vi "LP MDrive init.vi"(0 "VISA IN":refnum<visa-resource-name>="COM17", 1 "Factory Default":bool, 5 "error in":errorcluster, 6 "Hold Current":string="50", 7 "Accel Setpoint":string="300000", 8 "Working Velocity":string, 9 "Mdrive Mode":T1=enum."Party Mode", 11 "Device Name":string, 12 "Run Current":string="50", 13 "Decel Setpoint":string="300000") -> (14 "VISA OUT":refnum<visa-resource-name>="COM17", 19 "error out":errorcluster)   [LabVIEW 2015]
uses:
  MCode_LV_86/Set Parameter.ctl
  MCode_LV_86/Get Parameter.ctl
  MCode_LV_86/MDrive Mode.ctl
panel:
  out "read buffer":string
  out "OK":bool
  out "Error":string
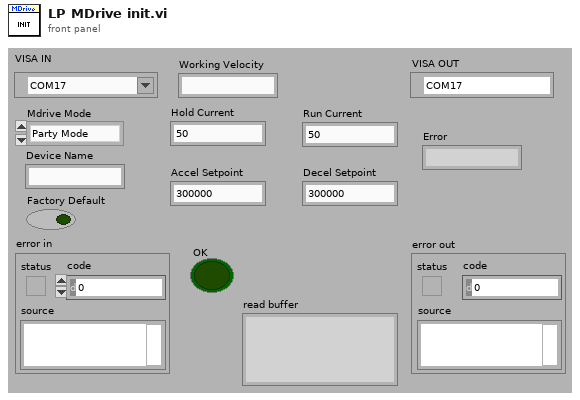
[diagram p1: front panel]
types:
  T1 = typedef "MDrive Mode.ctl" = enum16{"Normal Mode", "Party Mode"}
  T2 = typedef "Get Parameter.ctl" = enum16{"Acceleration (A)", "Baud Rate (BD)", "Busy Flag (BY)", "Counter 1 (C1)", "Counter 2 (C2)", "Check Sum Enable (CK)", "Clock Mode (CM)", "Clock Mode Ratio (CR)", "Clock Mode Out Step Width (CW)", "Deceleration (D)", "Digital Filtering, Input 1 (D1)", "Digital Filtering, Input 2 (D2)", "Digital Filtering, Input 3 (D3)", "Digital Filtering, Input 4 (D4)", "Digital Filtering, Input 5 (D5)", "Digital Filtering, Input 9 (D9)", "Digital Filtering, Input 10 (D10)", "Digital Filtering, Input 11 (D11)", "Digital Filtering, Input 12 (D12)", "Deadband (DB)", "Enable/Disable Drive (DE)", "Device Name (DN)", "End Program Execution (E)", "Encoder Function Enable (EE)", "Encoder Lines (EL)", "Error Flag (EF)", "Error Variable (ER)", "Echo Mode (EM)", "Escape (ES)", "Execute Program at Address (EX)", "Hold Current (HC)", "Hold Current Delay Time (HI)", "Input 1 (I1)", "Input 2 (I2)", "Input 3 (I3)", "Input 4 (I4)", "Input 5 Analog (I5)", "Input 6 Encoder Index (I6)", "Input 9 (I9)", "Input 10 (I10)", "Input 11 (I11)", "Input 12 (I12)", "Input Low Byte (1-4) (IL)", "Input High Byte (9-12) (IH)", "Inputs Total (1-4,9-12) (IN)", "Internal Temperature (IT)", "Jog Enable (JE)", "Limit Stop Mode (LM)", "MicroStepping Select (MS)", "Motor Settling Delay Time (MT)", "Moving Flag (MV)", "Output 1 (O1)", "Output 2 (O2)", "Output 3 (O3)", "Output 4 (O4)", "Output 9 (O9)", "Output 10 (O10)", "Output 11 (O11)", "Output 12 (O12)", "Output High Byte (9-12) (OH)", "Output Low Byte (1-4) (OL)", "Output Total (1-4 and 9-12) (OT)", "Position (P)", "Position Captured at Trip (PC)", "Position Maintenance (PM)", "Part Number (PN)", "Party Mode (PY)", "Register 1 (R1)", "Register 2 (R2)", "Register 3 (R3)", "Register 4 (R4)", "Run Current (RC)", "Serial Number (SN)", "Stall Flag (ST)", "Stall Factor (SF)", "Stall Mode Set (SM)", "User Variables (UV)", "Velocity (V)", "Velocity Changing Flag (VC)", "Velocity Initial (VI)", "Version, Firmware (VR)", "Velocity Maximum (VM)", "Read Input1", "Read Input2"}
  T3 = typedef "Set Parameter.ctl" = enum16{"Acceleration (A)", "Baud Rate (BD)", "Counter 1 (C1)", "Counter 2 (C2)", "Control C Software Reset (CE)", "Check Sum Enable (CK)", "Clock Mode (CM)", "Clock Mode Ratio (CR)", "Clock Mode Out Step Width (CW)", "Deceleration (D)", "Digital Filtering, Input 1 (D1)", "Digital Filtering, Input 2 (D2)", "Digital Filtering, Input 3 (D3)", "Digital Filtering, Input 4 (D4)", "Digital Filtering, Input 5 (D5)", "Digital Filtering, Input 9 (D9)", "Digital Filtering, Input 10 (D10)", "Digital Filtering, Input 11 (D11)", "Digital Filtering, Input 12 (D12)", "Deadband (DB)", "Decrement Variable (DC)", "Enable/Disable Drive (DE)", "Device Name (DN)", "End Program Execution (E)", "Encoder Function Enable (EE)", "Encoder Lines (EL)", "Echo Mode (EM)", "Error Clear (ER)", "Escape (ES)", "Execute Program at Address (EX)", "Factory Default (FD)", "Hold (H)", "Hold Current (HC)", "Hold Current Encoder Index (HI)", "Home to Home Switch (HM)", "Home to Delay Time (HT)", "Increment Variable (IC)", "Initialize Parameters to NVM (IP)", "Input into Variable (IV)", "Jog Enable (JE)", "Limit Stop Mode (LM)", "Move Absolute (MA)", "Move Relative (MR)", "MicroStepping Select (MS)", "Motor Settling Delay Time (MT)", "Output 1 (O1)", "Output 2 (O2)", "Output 3 (O3)", "Output 4 (O4)", "Output 9 (O9)", "Output 10 (O10)", "Output 11 (O11)", "Output 12 (O12)", "Output High Byte (9-12) (OH)", "Output Low Byte (1-4) (OL)", "Output Total (1-4 and 9-12) (OT)", "Position (P)", "Position Maintenance (PM)", "Party Mode (PY)", "Register 1 (R1)", "Register 2 (R2)", "Register 3 (R3)", "Register 4 (R4)", "Run Current (RC)", "Stall Factor (SF)", "Slew (SL)", "Stall Mode Set (SM)", "Upgrade Firmware (UG)", "Velocity Initial (VI)", "Velocity Maximum (VM)", "Set Input #1 as Home (S1)", "Save (S)", "Save DN+PY (NameS)", "Active Party Mode (0x0A)", "Set Input #1 (S1) as Limit- Active Floating", "Set Input #2 (S2) as Limit+ Active Floating", "Set Input #1 as Home (S1) Active Floating", "Set Input #1 as Home (S2) Active Floating", "Set Input #1 (S1) as Limit+ Active Floating", "Set Input #2 (S2) as Limit- Active Floating", "Hybrid Mode (AS)"}
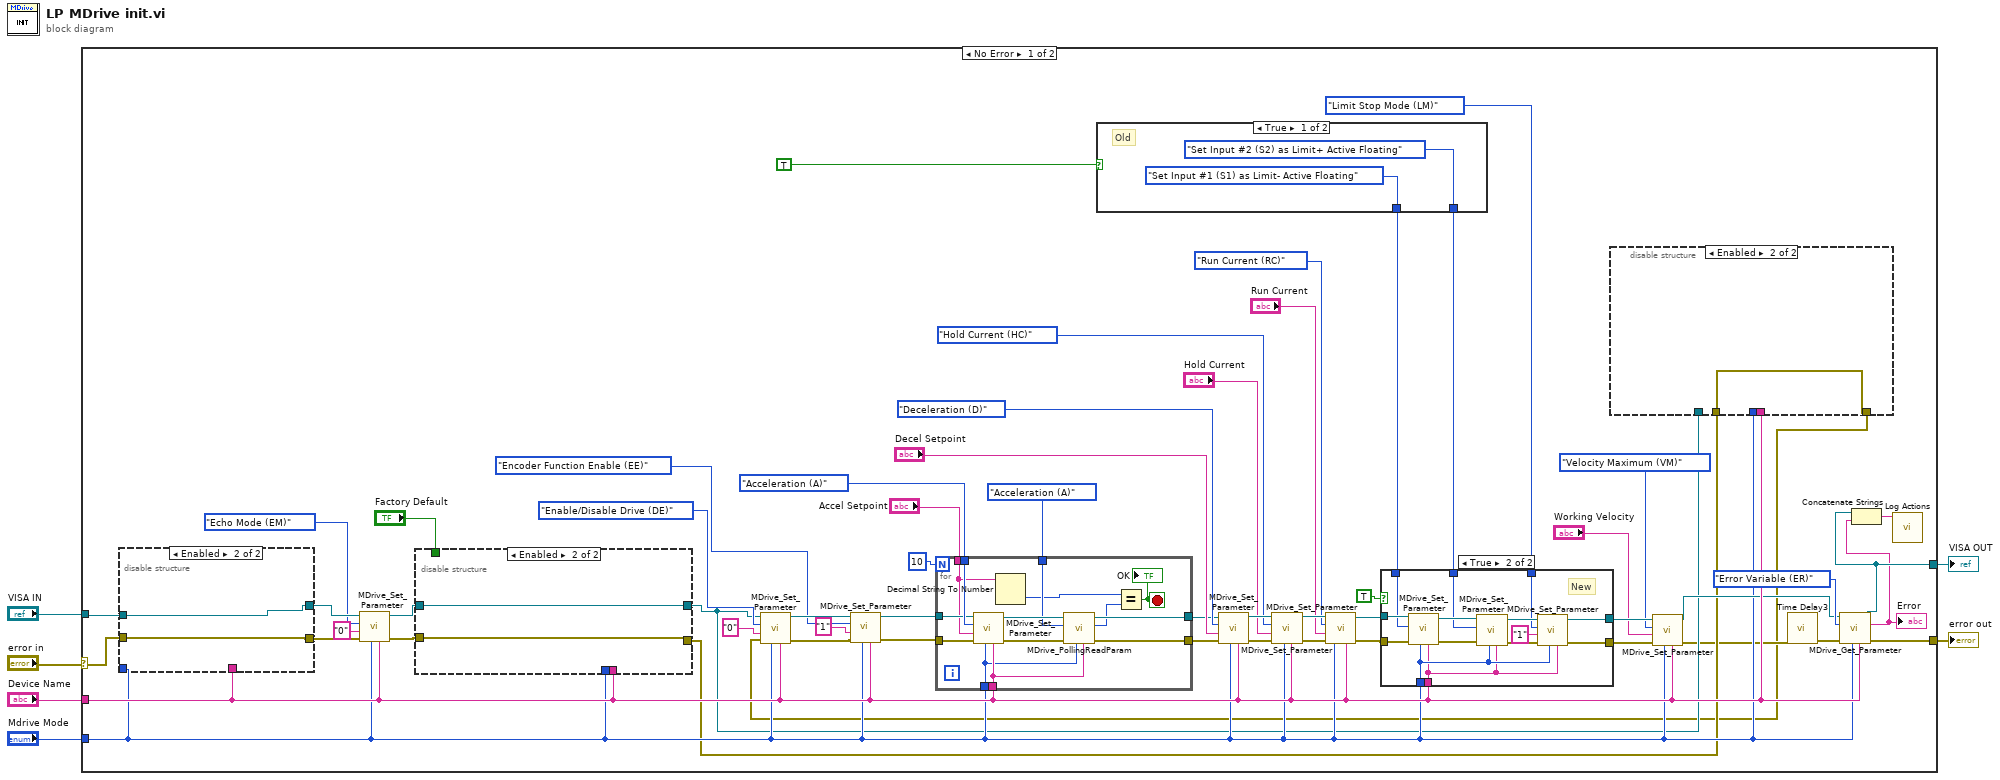
[diagram p0: block diagram]
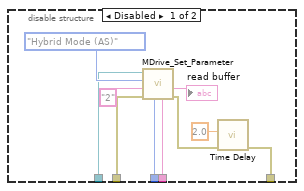
[diagram p2: hidden frame]
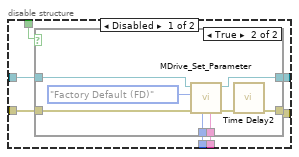
[diagram p3: hidden frame]
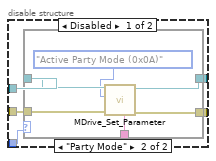
[diagram p5: hidden frame]
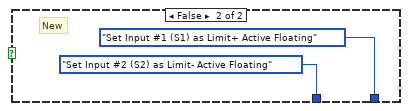
[diagram p7: hidden frame]
diagram:
  n1 = case shown="No Error" "error in" {
    selector: "error in" -> [w35 w145]
    tunnel: [w43 w144] -> w3
    tunnel: [w48 w145] -> w6
    tunnel: "VISA IN" -> [w36 w144]
    tunnel: "Device Name" -> [w13 _]
    tunnel: "Mdrive Mode" -> [w11 _]
    frame No Error {
      n2 = disable-structure shown="Enabled" {
        disable-tunnel: w36 -> [w113 w123]
        disable-tunnel: w35 -> [w112 w122]
        disable-tunnel: [w111 w123] -> w34
        disable-tunnel: [w110 w122] -> w33
        disable-tunnel: w13 -> [w109 _]
        disable-tunnel: w11 -> [w108 _]
        frame Disabled {
          n3 = case shown="\"Party Mode\"" w108 {
            tunnel: [w114 w121] -> w110
            tunnel: w112 -> [w114 w120]
            tunnel: [w115 w119] -> w111
            tunnel: w113 -> [w115 w118]
            tunnel: w109 -> [_ w116]
            frame "Normal Mode", Default {
            }
            frame "Party Mode" {
              n4 = call "MDrive_Set_Parameter.vi"("Device Name"=w116, "error in"=w120, "Set Parameter"=Set_Parameter."Active Party Mode (0x0A)", "VISA IN"=w118) -> ("error out"=w121:errorcluster, "VISA OUT"=w119:refnum<visa-resource-name>)  [unwired: 5 in, 1 out]
            }
          }
        }
        frame Enabled {
        }
      }
      n5 = call "MDrive_Set_Parameter.vi"("Device Name"=w13, "Mdrive Mode"=w11, "error in"=w33, "Parameter Setpoint"="0", "Set Parameter"=Set_Parameter."Echo Mode (EM)", "VISA IN"=w34) -> ("error out"=w32:errorcluster, "VISA OUT"=w31:refnum<visa-resource-name>)  [unwired: 3 in, 1 out]
      n6 = disable-structure shown="Enabled" {
        disable-tunnel: [w95 w106] -> w10
        disable-tunnel: [w94 w107] -> w9
        disable-tunnel: "Factory Default" -> [w93 _]
        disable-tunnel: w32 -> [w92 w106]
        disable-tunnel: w31 -> [w91 w107]
        disable-tunnel: w13 -> [w90 _]
        disable-tunnel: w11 -> [w89 _]
        frame Disabled {
          n7 = case shown="True" w93 {
            tunnel: [w96 w105] -> w95
            tunnel: w91 -> [w97 w104]
            tunnel: [w97 w103] -> w94
            tunnel: w92 -> [w96 w100]
            tunnel: w90 -> [_ w99]
            tunnel: w89 -> [_ w98]
            frame False {
            }
            frame True {
              n8 = call "MDrive_Set_Parameter.vi"("Device Name"=w99, "Mdrive Mode"=w98, "error in"=w100, "Set Parameter"=Set_Parameter."Factory Default (FD)", "VISA IN"=w104) -> ("error out"=w102:errorcluster, "VISA OUT"=w103:refnum<visa-resource-name>)  [unwired: 4 in, 1 out]
              n9 = call "Time Delay2"("error in (no error)"=w102) -> ("error out"=w105:errorcluster)  [unwired: 10 in]
            }
          }
        }
        frame Enabled {
        }
      }
      n10 = case shown="True" TRUE {
        tunnel: [Set_Parameter."Set Input #1 (S1) as Limit- Active Floating" ("Set Parameter") Set_Parameter."Set Input #2 (S2) as Limit- Active Floating" ("Set Parameter")] -> w41
        tunnel: [Set_Parameter."Set Input #2 (S2) as Limit+ Active Floating" ("Set Parameter") Set_Parameter."Set Input #1 (S1) as Limit+ Active Floating" ("Set Parameter")] -> w40
        frame True {
          # "Old"
        }
        frame False {
          # "New"
        }
      }
      n11 = disable-structure shown="Enabled" {
        disable-tunnel: w13 -> [w73 _]
        disable-tunnel: w11 -> [w72 _]
        disable-tunnel: w10 -> [w69 w74]
        disable-tunnel: w9 -> [w68 _]
        disable-tunnel: [w65 w74] -> w7
        frame Disabled {
          n12 = call "MDrive_Set_Parameter.vi"("Device Name"=w73, "Mdrive Mode"=w72, "error in"=w69, "Parameter Setpoint"="2", "Set Parameter"=Set_Parameter."Hybrid Mode (AS)", "VISA IN"=w68) -> ("error out"=w66:errorcluster, "read buffer"=→"read buffer":string)  [unwired: 3 in, 1 out]
          n13 = call "Time Delay"("error in (no error)"=w66, "Delay Time (s)"=2.0) -> ("error out"=w65:errorcluster)  [unwired: 9 in]
        }
        frame Enabled {
        }
      }
      n14 = call "MDrive_Set_Parameter.vi"("Device Name"=w13, "Mdrive Mode"=w11, "error in"=w7, "Parameter Setpoint"="0", "Set Parameter"=Set_Parameter."Enable/Disable Drive (DE)", "VISA IN"=w9) -> ("error out"=w17:errorcluster, "VISA OUT"=w18:refnum<visa-resource-name>)  [unwired: 3 in, 1 out]
      n15 = call "MDrive_Set_Parameter.vi"("Device Name"=w13, "Mdrive Mode"=w11, "error in"=w17, "Parameter Setpoint"="1", "Set Parameter"=Set_Parameter."Encoder Function Enable (EE)", "VISA IN"=w18) -> ("error out"=w16:errorcluster, "VISA OUT"=w15:refnum<visa-resource-name>)  [unwired: 3 in, 1 out]
      n16 = for {
        N: 10 -> [_]
        tunnel: "Accel Setpoint" -> [w77]
        tunnel: Set_Parameter."Acceleration (A)" ("Set Parameter") -> [w88]
        tunnel: w15 -> [w87]
        tunnel: w16 -> [w86]
        tunnel: [w83] -> w24
        tunnel: [w82] -> w23
        tunnel: Get_Parameter."Acceleration (A)" ("Get Parameter") -> [w81]
        tunnel: w13 -> [w80]
        tunnel: w11 -> [w79]
        stop <- w75 stop-if-true
        n17 = call "MDrive_Set_Parameter.vi"("Device Name"=w80, "Mdrive Mode"=w79, "error in"=w86, "Parameter Setpoint"=w77, "Set Parameter"=w88, "VISA IN"=w87) -> ("error out"=w84:errorcluster, "VISA OUT"=w85:refnum<visa-resource-name>)  [unwired: 3 in, 1 out]
        n18 = Decimal String To Number(string=w77) -> (number=w76:i32)  [unwired: 2 in, 1 out]
        n19 = call "MDrive_PollingReadParam.vi"("Device Name"=w80, "Mdrive Mode"=w79, "error in (no error)"=w84, "Get Parameter"=w81, "VISA Refnum in"=w85) -> ("error out"=w82:errorcluster, "Value"=w78:i32, "VISA Refnum out"=w83:refnum<visa-resource-name>)  [unwired: 3 in, 1 out]
        n20 = Equal?(x=w76, y=w78) -> (x = y?=w75:bool)
        "OK" <- w75
      }
      n21 = call "MDrive_Set_Parameter.vi"("Device Name"=w13, "Mdrive Mode"=w11, "error in"=w23, "Parameter Setpoint"="Decel Setpoint", "Set Parameter"=Set_Parameter."Deceleration (D)", "VISA IN"=w24) -> ("error out"=w60:errorcluster, "VISA OUT"=w61:refnum<visa-resource-name>)  [unwired: 3 in, 1 out]
      n22 = call "MDrive_Set_Parameter.vi"("Device Name"=w13, "Mdrive Mode"=w11, "error in"=w60, "Parameter Setpoint"="Hold Current", "Set Parameter"=Set_Parameter."Hold Current (HC)", "VISA IN"=w61) -> ("error out"=w58:errorcluster, "VISA OUT"=w59:refnum<visa-resource-name>)  [unwired: 3 in, 1 out]
      n23 = call "MDrive_Set_Parameter.vi"("Device Name"=w13, "Mdrive Mode"=w11, "error in"=w58, "Parameter Setpoint"="Run Current", "Set Parameter"=Set_Parameter."Run Current (RC)", "VISA IN"=w59) -> ("error out"=w19:errorcluster, "VISA OUT"=w20:refnum<visa-resource-name>)  [unwired: 3 in, 1 out]
      n24 = case shown="True" TRUE {
        tunnel: w20 -> [w129 w143]
        tunnel: w19 -> [w128 w142]
        tunnel: w11 -> [_ w131]
        tunnel: w13 -> [_ w130]
        tunnel: [w128 w134] -> w27
        tunnel: [w129 w135] -> w28
        tunnel: w41 -> [_ w139]
        tunnel: w40 -> [_ w138]
        tunnel: Set_Parameter."Limit Stop Mode (LM)" ("Set Parameter") -> [_ w133]
        frame False {
          # "OLD"
        }
        frame True {
          # "New"
          n25 = call "MDrive_Set_Parameter.vi"("Device Name"=w130, "Mdrive Mode"=w131, "error in"=w142, "Set Parameter"=w139, "VISA IN"=w143) -> ("error out"=w141:errorcluster, "VISA OUT"=w140:refnum<visa-resource-name>)  [unwired: 4 in, 1 out]
          n26 = call "MDrive_Set_Parameter.vi"("Device Name"=w130, "Mdrive Mode"=w131, "error in"=w141, "Set Parameter"=w138, "VISA IN"=w140) -> ("error out"=w137:errorcluster, "VISA OUT"=w136:refnum<visa-resource-name>)  [unwired: 4 in, 1 out]
          n27 = call "MDrive_Set_Parameter.vi"("Device Name"=w130, "Mdrive Mode"=w131, "error in"=w137, "Parameter Setpoint"="1", "Set Parameter"=w133, "VISA IN"=w136) -> ("error out"=w134:errorcluster, "VISA OUT"=w135:refnum<visa-resource-name>)  [unwired: 3 in, 1 out]
        }
      }
      n28 = call "MDrive_Set_Parameter.vi"("Device Name"=w13, "Mdrive Mode"=w11, "error in"=w27, "Parameter Setpoint"="Working Velocity", "Set Parameter"=Set_Parameter."Velocity Maximum (VM)", "VISA IN"=w28) -> ("error out"=w8:errorcluster, "VISA OUT"=w12:refnum<visa-resource-name>)  [unwired: 3 in, 1 out]
      n29 = call "Time Delay3"("error in (no error)"=w8) -> ("error out"=w49:errorcluster)  [unwired: 10 in]
      n30 = call "MDrive_Get_Parameter.vi"("Device Name"=w13, "Mdrive Mode"=w11, "error in"=w49, "Get Parameter"=Get_Parameter."Error Variable (ER)", "VISA IN"=w12) -> ("error out"=w48:errorcluster, "Parameter Data String"=w42:string, "VISA OUT"=w43:refnum<visa-resource-name>)  [unwired: 3 in, 1 out]
      "Error" <- w42
      n31 = Concatenate Strings(w43, w42) -> (w44:string)
      n32 = call "Log Actions.vi"("Action"=w44) -> ()  [unwired: 8 in, 3 out]
    }
    frame Error {
    }
  }
  "VISA OUT" <- w3
  "error out" <- w6
